vi "definitive001.vi"() -> ()   [LabVIEW 2011]
uses:
  <vilib>/DAQmx/write.llb/DAQmx Write (Digital 1D Bool 1Chan 1Samp).vi
  <vilib>/DAQmx/read.llb/DAQmx Read (Analog DBL 1Chan 1Samp).vi
  <vilib>/DAQmx/create/channels.llb/DAQmx Create Channel (AI-Voltage-Basic).vi
  <vilib>/DAQmx/create/channels.llb/DAQmx Create Channel (DO-Digital Output).vi
  <vilib>/DAQmx/miscellaneous.llb/DAQmx Fill In Error Info.vi
  <vilib>/vision/NI_Vision_Development_Module.lvlib
panel:
  out "data":dbl caption="Daten" format="%0.2f"
  out "Image":T1(plugin-control)
  in  "Stop (F)":bool
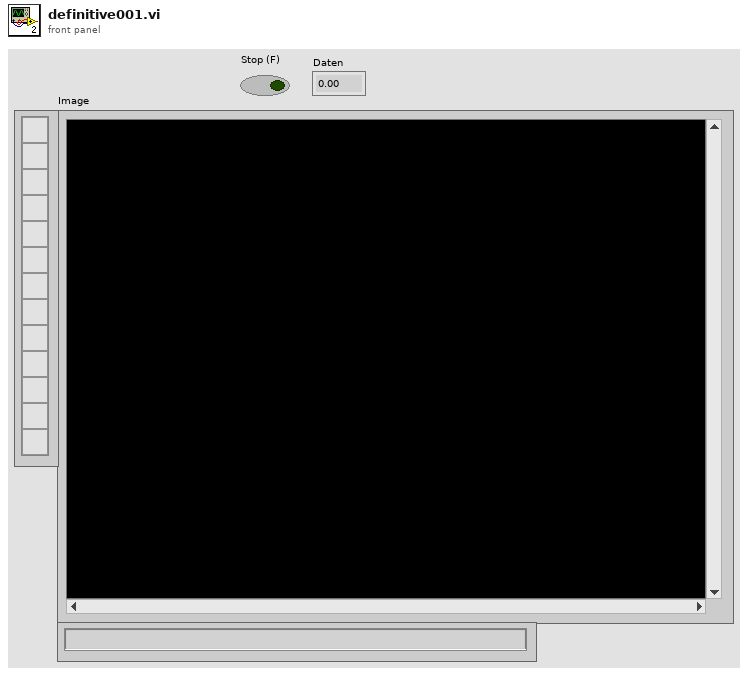
[diagram p1: front panel]
types:
  T1 = typedef "IMAQ Image.ctl" = refnum<image>
  T2 = cluster{"Position":cluster{"x":sgl, "y":sgl}, "Angle":sgl, "Scale":sgl, "Score":sgl, "Bounding Box":cluster{"x":sgl, "y":sgl}[]}[]
  T3 = cluster{"Matches (Pattern Matching 1)[0]":cluster{"Position":cluster{"x":sgl, "y":sgl}, "Angle":sgl, "Scale":sgl, "Score":sgl, "Bounding Box":cluster{"x":sgl, "y":sgl}[]}, "Matches (Pattern Matching 1)[1]":cluster{"Position":cluster{"x":sgl, "y":sgl}, "Angle":sgl, "Scale":sgl, "Score":sgl, "Bounding Box":cluster{"x":sgl, "y":sgl}[]}, "Matches (Pattern Matching 1)[2]":cluster{"Position":cluster{"x":sgl, "y":sgl}, "Angle":sgl, "Scale":sgl, "Score":sgl, "Bounding Box":cluster{"x":sgl, "y":sgl}[]}, "Matches (Pattern Matching 1)[3]":cluster{"Position":cluster{"x":sgl, "y":sgl}, "Angle":sgl, "Scale":sgl, "Score":sgl, "Bounding Box":cluster{"x":sgl, "y":sgl}[]}, "Matches (Pattern Matching 1)[4]":cluster{"Position":cluster{"x":sgl, "y":sgl}, "Angle":sgl, "Scale":sgl, "Score":sgl, "Bounding Box":cluster{"x":sgl, "y":sgl}[]}, "Matches (Pattern Matching 1)[5]":cluster{"Position":cluster{"x":sgl, "y":sgl}, "Angle":sgl, "Scale":sgl, "Score":sgl, "Bounding Box":cluster{"x":sgl, "y":sgl}[]}, "Matches (Pattern Matching 1)[6]":cluster{"Position":cluster{"x":sgl, "y":sgl}, "Angle":sgl, "Scale":sgl, "Score":sgl, "Bounding Box":cluster{"x":sgl, "y":sgl}[]}, "Matches (Pattern Matching 1)[7]":cluster{"Position":cluster{"x":sgl, "y":sgl}, "Angle":sgl, "Scale":sgl, "Score":sgl, "Bounding Box":cluster{"x":sgl, "y":sgl}[]}, "Matches (Pattern Matching 1)[8]":cluster{"Position":cluster{"x":sgl, "y":sgl}, "Angle":sgl, "Scale":sgl, "Score":sgl, "Bounding Box":cluster{"x":sgl, "y":sgl}[]}}
  T4 = cluster{"Matches (Pattern Matching 1)[0]":cluster{"Position":cluster{"x":sgl, "y":sgl}, "Angle":sgl, "Scale":sgl, "Score":sgl, "Bounding Box":cluster{"x":sgl, "y":sgl}[]}, "Matches (Pattern Matching 1)[1]":cluster{"Position":cluster{"x":sgl, "y":sgl}, "Angle":sgl, "Scale":sgl, "Score":sgl, "Bounding Box":cluster{"x":sgl, "y":sgl}[]}, "Matches (Pattern Matching 1)[2]":cluster{"Position":cluster{"x":sgl, "y":sgl}, "Angle":sgl, "Scale":sgl, "Score":sgl, "Bounding Box":cluster{"x":sgl, "y":sgl}[]}, "Matches (Pattern Matching 1)[3]":cluster{"Position":cluster{"x":sgl, "y":sgl}, "Angle":sgl, "Scale":sgl, "Score":sgl, "Bounding Box":cluster{"x":sgl, "y":sgl}[]}}
  T5 = cluster{"Bounding Box[0]":cluster{"x":sgl, "y":sgl}, "Bounding Box[1]":cluster{"x":sgl, "y":sgl}, "Bounding Box[2]":cluster{"x":sgl, "y":sgl}, "Bounding Box[3]":cluster{"x":sgl, "y":sgl}}
  T6 = cluster{"[0]":sgl, "[1]":sgl, "[2]":sgl, "[3]":sgl}
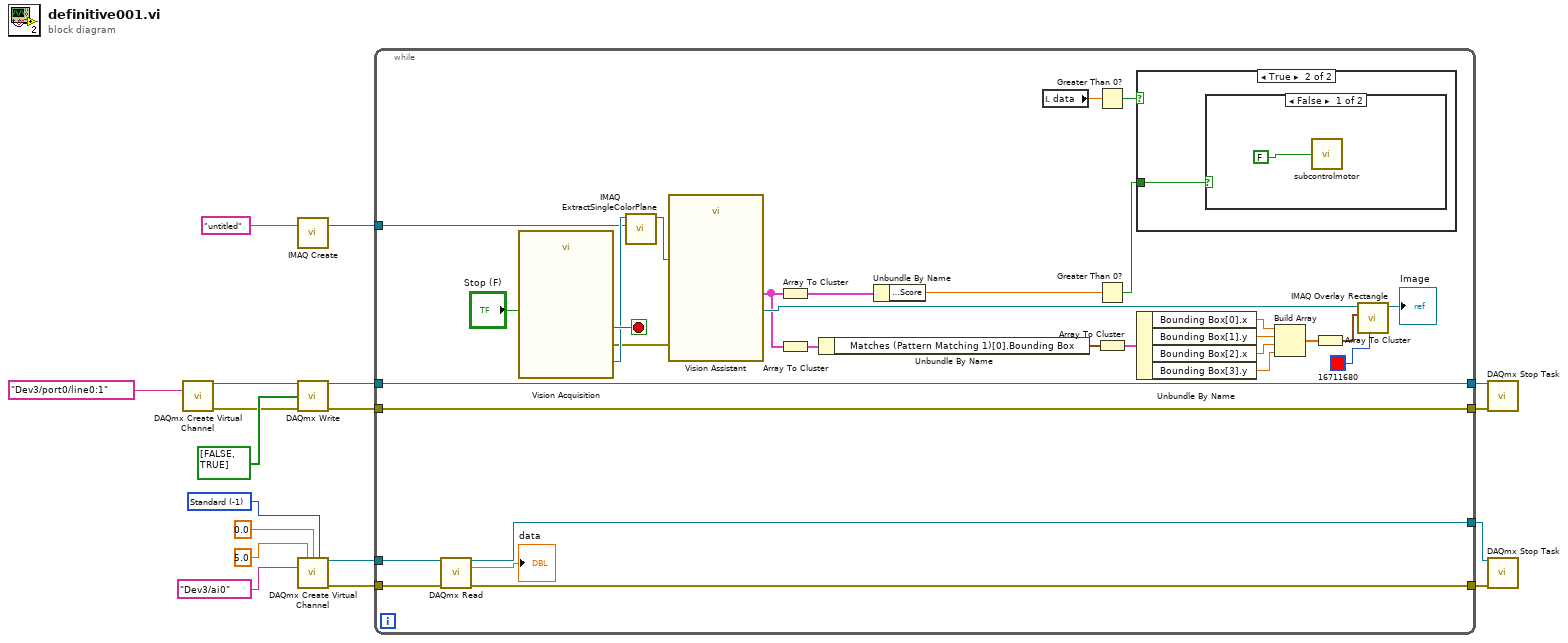
[diagram p0: block diagram]
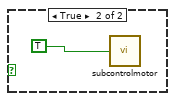
[diagram p3: hidden frame]
diagram:
  w13 = -1 items=["Standard"=-1, "RSE"=10083, "NRSE"=10078, "Differentiell"=10106, "Pseudodifferentiell"=12529] ("input terminal configuration")
  n1 = call-poly <vilib>:"DAQmx Create Virtual Channel.vi"("lines"=tag "Dev3/port0/line0:1") -> ("task out"=w4:refnum<k21>, "error out"=w3:errorcluster)  [unwired: 13 in]
  n2 = call "IMAQ Create"("Image Name"="untitled") -> ("New Image"=w17:T1)  [unwired: 4 in, 1 out]
  n3 = call-poly <vilib>:"DAQmx Write.vi"("task/channels in"=w4, "data"=bool[] [FALSE, TRUE], "error in"=w3) -> ("task out"=w2:refnum<k21>, "error out"=w1:errorcluster)  [unwired: 10 in, 1 out]
  n4 = call-poly <vilib>:"DAQmx Create Virtual Channel.vi"("maximum value"=5.0, "minimum value"=0.0, "input terminal configuration"=w13, "physical channels"=tag "Dev3/ai0") -> ("task out"=w12:refnum<k21>, "error out"=w11:errorcluster)  [unwired: 10 in]
  n5 = while {
    tunnel: w17 -> [w46]
    tunnel: w12 -> [w27]
    tunnel: w11 -> [w26]
    tunnel: [w25] -> w10
    tunnel: [w24] -> w9
    tunnel: [w20] -> w7
    tunnel: [w19] -> w6
    tunnel: w2 -> [w20]
    tunnel: w1 -> [w19]
    stop <- w48 stop-if-true
    n6 = call-poly <vilib>:"DAQmx Read.vi"("task/channels in"=w27, "error in"=w26) -> ("task out"=w25:refnum<k21>, "data"=→"data":dbl, "error out"=w24:errorcluster)  [unwired: 11 in]
    n7 = call "Vision Acquisition"("Stop (F)"="Stop (F)") -> ("Image Out"=w47:T1, "Stopped"=w48:bool, "error out"=w45:errorcluster)  [unwired: 24 in]
    n8 = call "IMAQ ExtractSingleColorPlane"("Image Dst"=w46, "Image Src"=w47) -> ("Image Dst Out"=w44:T1)  [unwired: 8 in, 1 out]
    n9 = call "Vision Assistant"("Image In"=w44, "error in"=w45) -> ("Image Out"=w34:T1, "Matches (Pattern Matching 1)"=w31:T2)  [unwired: 23 in, 1 out]
    n10 = Array To Cluster(array=w31) -> (cluster=w30:T3)
    n11 = Array To Cluster(array=w31) -> (cluster=w43:T4)
    n12 = Unbundle By Name(w43) -> ("Matches (Pattern Matching 1)[0].Bounding Box"=w42:cluster{"x":sgl, "y":sgl}[])
    n13 = Unbundle By Name(w30) -> ("Matches (Pattern Matching 1)[0].Score"=w29:sgl)
    n14 = local read "data"() -> (w23:dbl)
    n15 = Greater Than 0?(x=w23) -> (x > 0?=w22:bool)
    n16 = Greater Than 0?(x=w29) -> (x > 0?=w21:bool)
    n17 = Array To Cluster(array=w42) -> (cluster=w41:T5)
    n18 = case shown="True" w22 {
      tunnel: w21 -> [_ w50]
      frame False {
      }
      frame True {
        n19 = case shown="False" w50 {
          frame False {
            n20 = call "subcontrolmotor.vi"("Boolesch"=FALSE) -> ()
          }
          frame True {
            n21 = call "subcontrolmotor.vi"("Boolesch"=TRUE) -> ()
          }
        }
      }
    }
    n22 = Unbundle By Name(w41) -> ("Bounding Box[0].x"=w40:sgl, "Bounding Box[1].y"=w39:sgl, "Bounding Box[2].x"=w38:sgl, "Bounding Box[3].y"=w37:sgl)
    n23 = Build Array(w40, w39, w38, w37) -> (w36:sgl[])
    n24 = Array To Cluster(array=w36) -> (cluster=w35:T6)
    n25 = call "IMAQ Overlay Rectangle"("Color"=u32 16711680, "Rectangle"=w35, "Image"=w34) -> ("Image Out"=→"Image":T1)  [unwired: 7 in, 1 out]
  }
  n26 = call <vilib>:"DAQmx Stop Task.vi"("task/channels in"=w7, "error in"=w6) -> ()  [unwired: 12 in, 2 out]
  n27 = call <vilib>:"DAQmx Stop Task.vi"("task/channels in"=w10, "error in"=w9) -> ()  [unwired: 12 in, 2 out]
